vi "Simple Reader.vi"(8 "error in (no error)":errorcluster, 11 "Quantum Design Driver in":refnum<class "Quantum Design Driver.lvclass">) -> (0 "error out":errorcluster, 2 "Signals":dbl[](array[numeric]), 3 "Quantum Design Driver out":refnum<class "Quantum Design Driver.lvclass">)   [LabVIEW 2021, in "Quantum Design Driver.lvclass"]
uses:
  Quantum Design Driver.lvclass
  Quantum Design Driver.lvclass/Quantum Design Driver.ctl
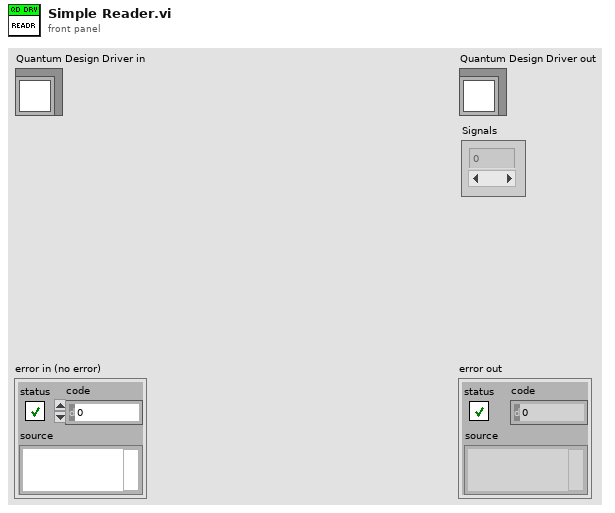
[diagram p1: front panel]
types:
  T1 = typedef "Quantum Desing Configuration.ctl" = cluster{"Address":string, "Instrument type":u16, "Remote":bool, "Measurements":enum16{"Temperature", "Field", "Position"}[]}
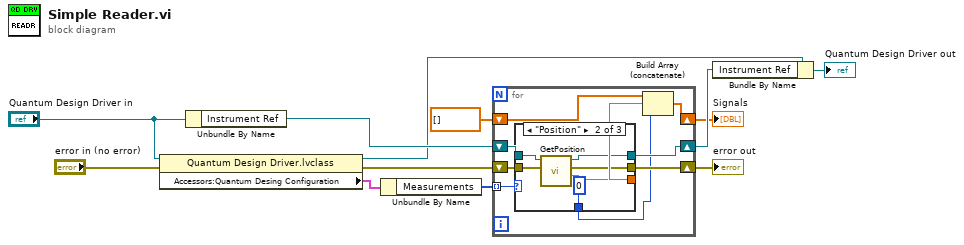
[diagram p0: block diagram]
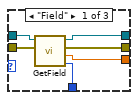
[diagram p2: hidden frame]
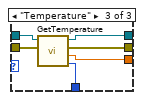
[diagram p3: hidden frame]
diagram:
  n1 = property class="Quantum Design Driver.lvclass"(reference="Quantum Design Driver in", error in="error in (no error)") -> (reference out=w8:refnum<class "Quantum Design Driver.lvclass">, error out=w5:errorcluster, "Accessors:Quantum Desing Configuration"=w11:T1)
  n2 = Unbundle By Name("Quantum Design Driver in") -> ("Instrument Ref"=w10:refnum<k24>)
  n3 = Unbundle By Name(w11) -> ("Measurements"=w6:enum16{"Temperature", "Field", "Position"}[])
  n4 = for {
    tunnel: w6 -> [w17] mode=indexing
    shift-right: [w14] -> w1
    shift-left: dbl[] [] -> [w16]
    shift-right: [w18] -> w3
    shift-left: w5 -> [w21]
    shift-right: [w19] -> w4
    shift-left: w10 -> [w20]
    n5 = case shown="\"Position\"" w17 {
      tunnel: w21 -> [w27 w33 w39]
      tunnel: w20 -> [w26 w32 w38]
      tunnel: [w25 w31 w37] -> w19
      tunnel: [w24 w30 w36] -> w18
      tunnel: [w23 w29 w35] -> w15
      tunnel: [w22 0 ("Field\nStatus") w34] -> w13
      frame "Field" {
        n6 = call <instrlib>:"GetField.vi"("error in (no error)"=w27, "Instrument Ref In"=w26) -> ("Field\nStatus"=w22:i32, "Field"=w23:dbl, "error out"=w24:errorcluster, "Instrument Ref Out"=w25:refnum<k24>)  [unwired: 3 in, 1 out]
      }
      frame "Position" {
        n7 = call <instrlib>:"GetPosition.vi"("error in (no error)"=w33, "Instrument Ref In"=w32) -> ("Position"=w29:dbl, "error out"=w30:errorcluster, "Instrument Ref Out"=w31:refnum<k24>)  [unwired: 2 in, 1 out]
      }
      frame "Temperature" {
        n8 = call <instrlib>:"GetTemperature.vi"("error in (no error)"=w39, "Instrument Ref In"=w38) -> ("Temperature\nStatus"=w34:i32, "Temperature"=w35:dbl, "error out"=w36:errorcluster, "Instrument Ref Out"=w37:refnum<k24>)  [unwired: 3 in, 1 out]
      }
    }
    n9 = Build Array (concatenate)(w16, w15, w13) -> (w14:dbl[])
  }
  "error out" <- w3
  "Signals" <- w1
  n10 = Bundle By Name(cluster=w8, "Instrument Ref"=w4) -> (→"Quantum Design Driver out":refnum<class "Quantum Design Driver.lvclass">)
